vi "Create Dynamical Model.vi"() -> ()   [LabVIEW 2020]
uses:
  Infrastructure/Dynamical System Model Definition.ctl
  Infrastructure/Model Types.ctl
panel:
  out "XY-Limited Robot Dynamical System Model":T1
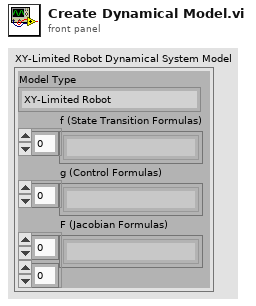
[diagram p1: front panel]
types:
  T1 = typedef "Dynamical System Model Definition.ctl" = cluster{"Model Type":T2, "f (State Transition Formulas)":string[], "g (Control Formulas)":string[], "F (Jacobian Formulas)":string[][]}
  T2 = typedef "Model Types.ctl" = enum16{"XY-Limited Robot", "Holonomic Robot (Acceleration Controlled)"}
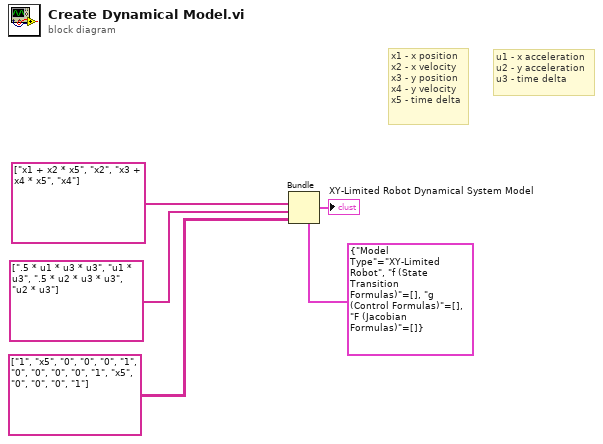
[diagram p0: block diagram]
diagram:
  # "u1 - x acceleration\nu2 - y acceleration\nu3 - time delta"
  # "x1 - x position\nx2 - x velocity\nx3 - y position\nx4 - y velocity\nx5 - time delta"
  n1 = Bundle(cluster=T1 {"Model Type"=enum."XY-Limited Robot", "f (State Transition Formulas)"=[], "g (Control Formulas)"=[], "F (Jacobian Formulas)"=[]} ("Dynamical System Model Definition"), "f (State Transition Formulas)"=string[] ["x1 + x2 * x5", "x2", "x3 + x4 * x5", "x4"], "g (Control Formulas)"=string[] [".5 * u1 * u3 * u3", "u1 * u3", ".5 * u2 * u3 * u3", "u2 * u3"], "F (Jacobian Formulas)"=string[][] [["1", "x5", "0", "0"], ["0", "1", "0", "0"], ["0", "0", "1", "x5"], ["0", "0", "0", "1"]]) -> (→"XY-Limited Robot Dynamical System Model":T1)  [unwired: 1 in]
